vi "Scale Byte Log.vi"(9 "Brightness":u8, 10 "Factor":dbl, 11 "Color":u8) -> (3 "Color Scaled":u8)   [LabVIEW 2013]
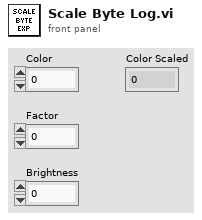
[diagram p1: front panel]
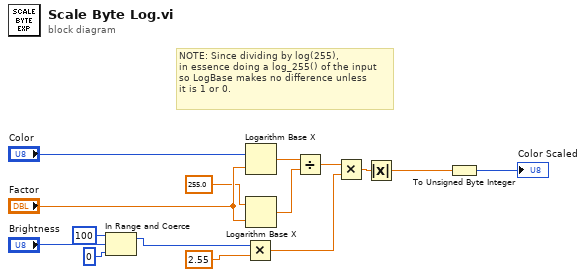
[diagram p0: block diagram]
diagram:
  # "NOTE: Since dividing by log(255),\nin essence doing a log_255() of the input\nso LogBase makes no difference unless\nit is 1 or 0."
  n1 = In Range and Coerce(upper limit=u8 100, x="Brightness", lower limit=u8 0) -> (coerced(x)=w3:u8)  [unwired: 1 out]
  n2 = Multiply(x=w3, y=2.55) -> (x*y=w13:dbl)
  n3 = Logarithm Base X(1:"Factor", 2:"Color") -> (0:w14:dbl)
  n4 = Logarithm Base X(1:"Factor", 2:255.0 ("y")) -> (0:w15:dbl)
  n5 = Divide(x=w14, y=w15) -> (x/y=w11:dbl)
  n6 = Multiply(x=w11, y=w13) -> (x*y=w12:dbl)
  n7 = Absolute Value(x=w12) -> (abs(x)=w2:dbl)
  n8 = To Unsigned Byte Integer(number=w2) -> (unsigned 8bit integer=→"Color Scaled":u8)
